vi "New GPS on GIC A.vi"(11 "GIC Input":T1={"     Use ?\nOff       On"=[FALSE, TRUE, FALSE, TRUE], "Mode:"=FALSE, "Rx Prop Port"="", "Hokuyo Port"="COM7", "Tx Prop  Port"="COM6", "Compass Port"="", "GPS Port"="", "Num of WPs"=0, "WP Lats and Longs"={"WP Lats"=[], "WP Longs"=[]}, "Obst Lats and Longs"={"Obst Lats"=[], "Obst Longs"=[]}, "Parameters"=[], "GPS Data"=[], "Compass"=0.0, "LMS Vector"=[], "Vision Vector"=[], "Direction Cmd"=0.0, "Speed Cmd"=0.0, "WP Vector"=[], "WP Number"=0, "Extra"=0, "SW Map"=[], "Path Cluster"={"Path x node"=[], "Path y node"=[]}} {"Obst Lats and Longs"."Obst Longs" format="%#_8g"; "Obst Lats and Longs"."Obst Lats" format="%#_8g"}) -> (3 "GIC Output":T1={"     Use ?\nOff       On"=[FALSE, TRUE, FALSE, TRUE], "Mode:"=FALSE, "Rx Prop Port"="", "Hokuyo Port"="COM7", "Tx Prop  Port"="COM6", "Compass Port"="", "GPS Port"="", "Num of WPs"=0, "WP Lats and Longs"={"WP Lats"=[], "WP Longs"=[]}, "Obst Lats and Longs"={"Obst Lats"=[], "Obst Longs"=[]}, "Parameters"=[], "GPS Data"=[], "Compass"=0.0, "LMS Vector"=[], "Vision Vector"=[], "Direction Cmd"=0.0, "Speed Cmd"=0.0, "WP Vector"=[], "WP Number"=0, "Extra"=0, "SW Map"=[], "Path Cluster"={"Path x node"=[], "Path y node"=[]}} {"Obst Lats and Longs"."Obst Longs" format="%#_8g"; "Obst Lats and Longs"."Obst Lats" format="%#_8g"})   [LabVIEW 2014]
panel:
  # "New GPS on GIC A"
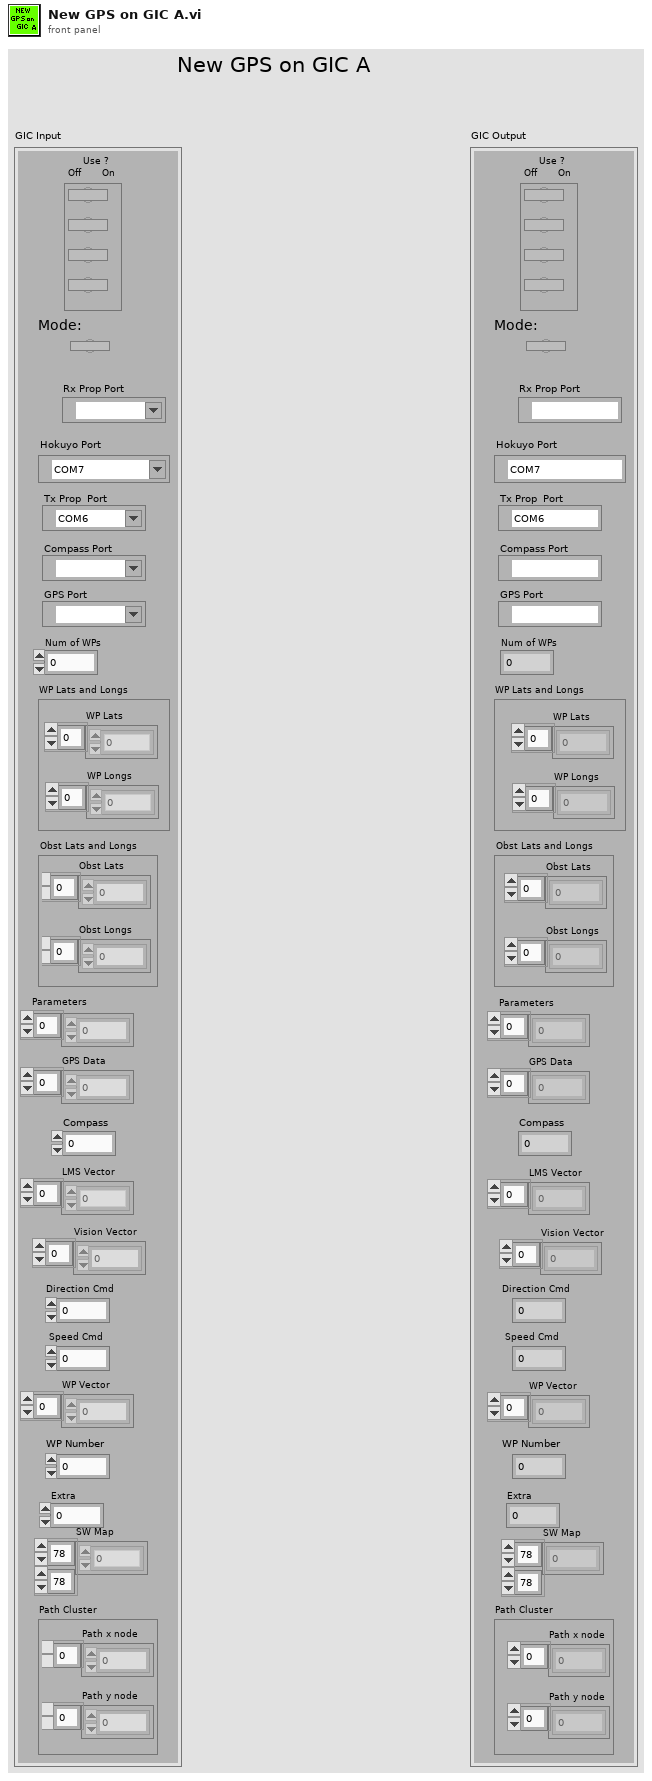
[diagram p1: front panel]
types:
  T1 = cluster{"     Use ?\nOff       On":bool[], "Mode:":bool, "Rx Prop Port":refnum<visa-resource-name>, "Hokuyo Port":refnum<visa-resource-name>, "Tx Prop  Port":refnum<visa-resource-name>, "Compass Port":refnum<visa-resource-name>, "GPS Port":refnum<visa-resource-name>, "Num of WPs":i16, "WP Lats and Longs":cluster{"WP Lats":dbl[], "WP Longs":dbl[]}, "Obst Lats and Longs":cluster{"Obst Lats":dbl[], "Obst Longs":dbl[]}, "Parameters":dbl[], "GPS Data":dbl[], "Compass":dbl, "LMS Vector":dbl[], "Vision Vector":dbl[], "Direction Cmd":dbl, "Speed Cmd":dbl, "WP Vector":dbl[], "WP Number":i32, "Extra":i16, "SW Map":i32[][], "Path Cluster":cluster{"Path x node":dbl[], "Path y node":dbl[]}}
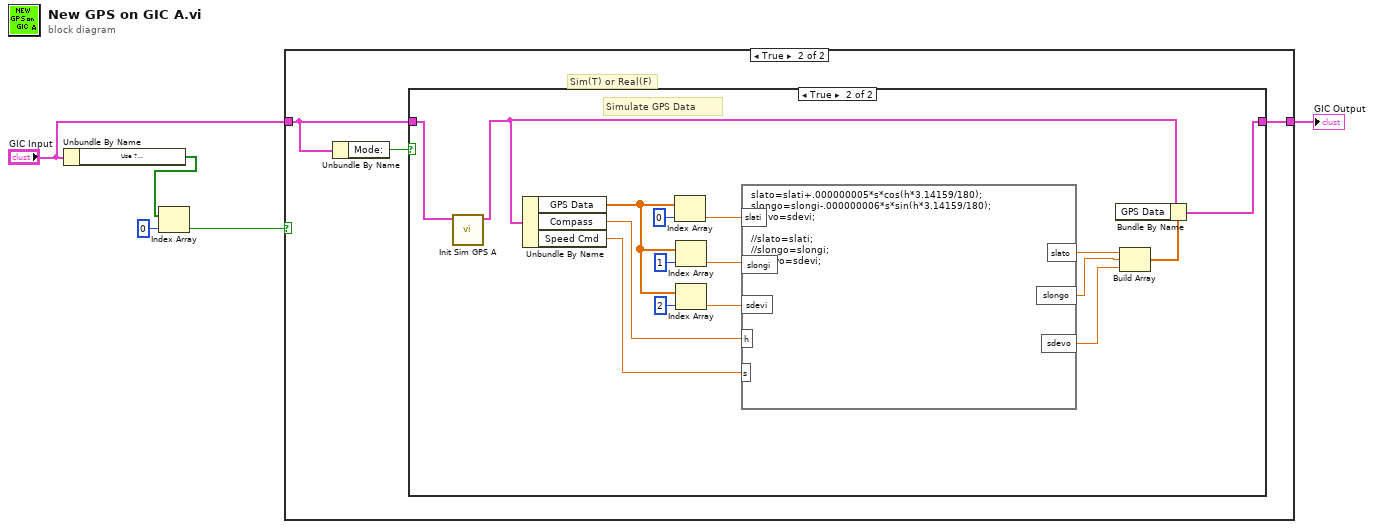
[diagram p0: block diagram]
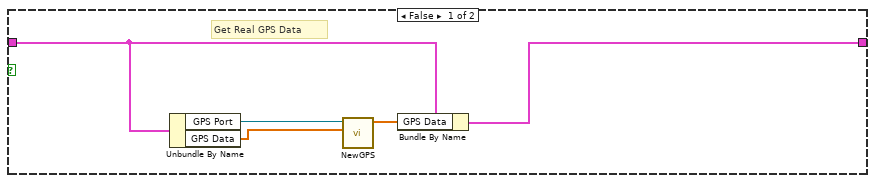
[diagram p3: hidden frame]
diagram:
  n1 = Unbundle By Name("GIC Input") -> ("Use ?\nOff       On"=w5:bool[])
  n2 = Index Array(array=w5, index=0) -> (element=w3:bool)
  n3 = case shown="True" w3 {
    tunnel: "GIC Input" -> [w6 w8]
    tunnel: [w6 w7] -> w1
    frame False {
    }
    frame True {
      # "Sim(T) or Real(F)"
      n4 = Unbundle By Name(w8) -> ("Mode:"=w9:bool)
      n5 = case shown="True" w9 {
        tunnel: w8 -> [w12 w16]
        tunnel: [w10 w17] -> w7
        frame False {
          # "Get Real GPS Data"
          n6 = Unbundle By Name(w12) -> ("GPS Port"=w14:refnum<visa-resource-name>, "GPS Data"=w13:dbl[])
          n7 = call "NewGPS.vi"("Input lat, long, dev"=w13, "GPS Com Port"=w14) -> ("Output lat, long, dev"=w11:dbl[])  [unwired: 9 in]
          n8 = Bundle By Name(cluster=w12, "GPS Data"=w11) -> (w10:T1)
        }
        frame True {
          # "Simulate GPS Data"
          n9 = call "Init Sim GPS A.vi"("GIC Input"=w16) -> ("GIC Output"=w15:T1)  [unwired: 10 in]
          n10 = Unbundle By Name(w15) -> ("GPS Data"=w26:dbl[], "Compass"=w23:dbl, "Speed Cmd"=w22:dbl)
          n11 = Index Array(array=w26, index=0) -> (element=w30:dbl)
          n12 = Index Array(array=w26, index=1) -> (element=w28:dbl)
          n13 = Index Array(array=w26, index=2) -> (element=w25:dbl)
          n14 = formula code="slato=slati+.000000005*s*cos(h*3.14159/180);\nslongo=slongi-.000000006*s*sin(h*3.14159/180);\nsdevo=sdevi;\n\n//slato=slati;\n//slongo=slongi;\n//sdevo=sdevi;"("slati"=w30, "slongi"=w28, "sdevi"=w25, "h"=w23, "s"=w22) -> ("slato"=w21:dbl, "slongo"=w20:dbl, "sdevo"=w19:dbl)
          n15 = Build Array(w21, w20, w19) -> (w18:dbl[])
          n16 = Bundle By Name(cluster=w15, "GPS Data"=w18) -> (w17:T1)
        }
      }
    }
  }
  "GIC Output" <- w1
